vi "write.vi"(7 "command":u8[](array[numeric]) format="%.0x", 8 "error in (no error)":errorcluster caption="错误输入（无错误）", 9 "count":i32, 11 "handle":u64) -> (0 "error out":errorcluster caption="错误输出", 1 "function return":i32, 3 "handle out":u64)   [LabVIEW 2018, in "InstrumentsPlayground.lvlib"]
doc: "CLIFFAPI int write(FT_HANDLE handle, uchar *data, int count);"
uses:
  InstrumentsPlayground.lvlib
panel:
  out "command 2":u8[](array[numeric]) format="%.0x"
  in  "data":string
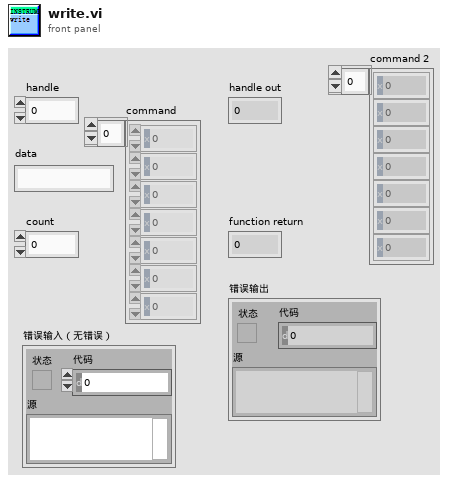
[diagram p1: front panel]
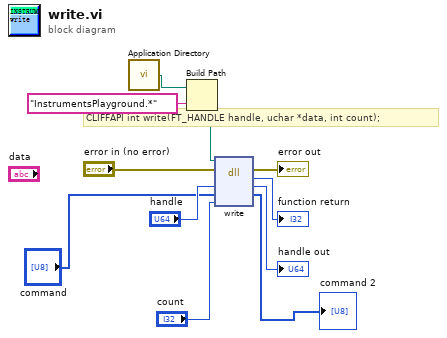
[diagram p0: block diagram]
diagram:
  # "CLIFFAPI int write(FT_HANDLE handle, uchar *data, int count);"
  n1 = call <vilib>:"Application Directory.vi"() -> ("Application Directory"=w4:path)
  n2 = Build Path(base path=w4, name or relative path="InstrumentsPlayground.*" ("名称或相对路径")) -> (appended path=w3:path)
  n3 = dll-call lib="E:/work/YZCourse_Xtext/Cliff/API/IPLabView lib/InstrumentsPlayground.*" fn="write"(path in=w3, error in="error in (no error)", "handle"="handle", "data"="command", "count"="count") -> (error out=→"error out":errorcluster, "返回类型"=→"function return":i32, "handle"=→"handle out":u32, "data"=→"command 2":u8[])  [unwired: 2 in, 1 out]
